vi "Moving Speed.vi"(8 "error in (no error)":errorcluster, 11 "Speed":dbl[](array[numeric])) -> (0 "error out":errorcluster)   [LabVIEW 2011]
panel:
  in  "VISA resource name":refnum<visa-resource-name>
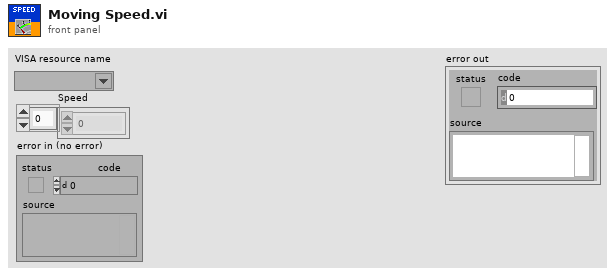
[diagram p1: front panel]
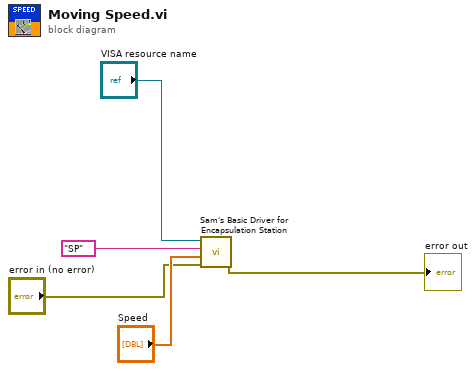
[diagram p0: block diagram]
diagram:
  n1 = call "Sam's Basic Driver for Encapsulation Station.vi"("error in (no error)"="error in (no error)", "Parameter Array"="Speed", "Combo Box"="SP", "VISA resource name"="VISA resource name") -> ("error out"=→"error out":errorcluster)  [unwired: 5 in, 2 out]
